vi "BattlesonEXC3t1.vi"() -> ()   [LabVIEW 2014, in "Battleson_Robot_12-2-16.lvrbt"]
uses:
  C:/Users/blb1094/Documents/LabVIEW Data/NXTRobotics/Projects/Battleson_Robot_12-2-16/Battleson_Robot_12-2-16.lvrbt
  <vilib>/NXT/Dual Mode Library/Sensors/EV3_Ultrasonic_CM.vi
  <vilib>/NXT/Dual Mode Library/Display/drawText_Center.vi
panel:
  in  "stop":bool
  out "wall proximity":string
  out "distance LED":bool
  out "current distance":dbl
  in  "min distance":dbl
  in  "max distance":dbl
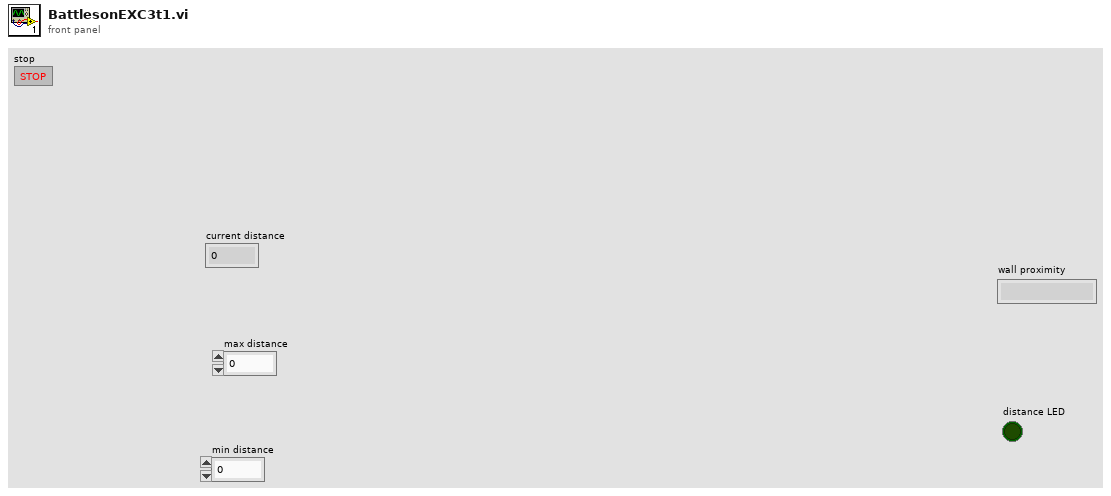
[diagram p1: front panel]
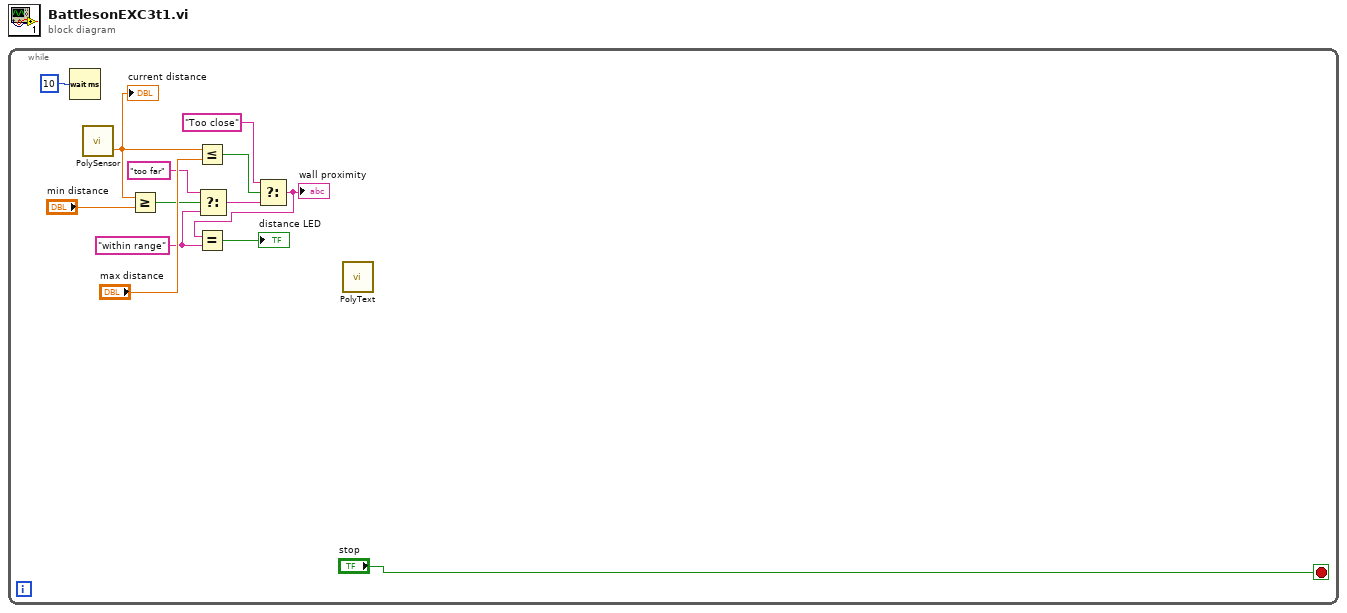
[diagram p0: block diagram]
diagram:
  n1 = while {
    stop <- "stop" stop-if-true
    w2 = "within range"
    n2 = Wait (ms)(milliseconds to wait=u32 10) -> ()  [unwired: 1 out]
    n3 = call-poly <vilib>:"PolySensor.vi"() -> ("Centimeters"=w13:sgl)  [unwired: 3 in, 1 out]
    "current distance" <- w13
    n4 = Greater Or Equal?(x=w13, y="min distance") -> (x >= y?=w10:bool)
    n5 = Less Or Equal?(x=w13, y="max distance") -> (x <= y?=w5:bool)
    n6 = Select(t="too far", s=w10, f=w2) -> (s? t:f=w9:string)
    n7 = Select(t="Too close", s=w5, f=w9) -> (s? t:f=w1:string)
    "wall proximity" <- w1
    n8 = Equal?(x=w1, y=w2) -> (x = y?=→"distance LED":bool)
    n9 = call-poly <vilib>:"PolyText.vi"() -> ()  [unwired: 4 in, 1 out]
  }
